vi "gGeneral.vi"() -> ()   [LabVIEW 2019]
panel:
  in  "Global Quit":bool
  in  "Plot Buffer Size":u8=5 max=10
  in  "Buffer Size":u8=100
  in  "Master Initialization?":bool=TRUE
  in  "Global Cancel":bool
  # "General Global Controls"
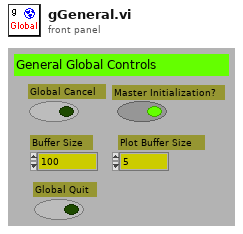
[diagram p1: front panel]
diagram:
